vi "Configure Route Marker Signal.vi"(8 "error in (no error)":errorcluster, 10 "Route Marker Signal (0: M1)":i32(ring) items=["Marker 1", "Marker 2", "Marker 3", "Marker 4", "AUX29", "None"], 11 "VISA resource name":refnum<visa-resource-name>) -> (0 "error out":errorcluster, 3 "VISA resource name out":refnum<visa-resource-name>)   [LabVIEW 2018, in "Agilent PSG MXG Series.lvlib"]
doc: "Configures the marker single to be routed to the rear panel EVENT 1 connector.\n\n<b>Note:</b>\nIt is applicable for N5172B with <b>Option 653 or <b>Option 655</b>, N5182B with <b>Option 656</b> or <b>Option 657</b> only."
uses:
  Agilent PSG MXG Series.lvlib
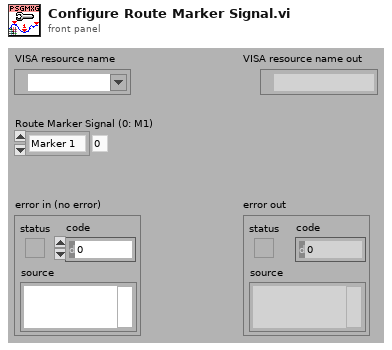
[diagram p1: front panel]
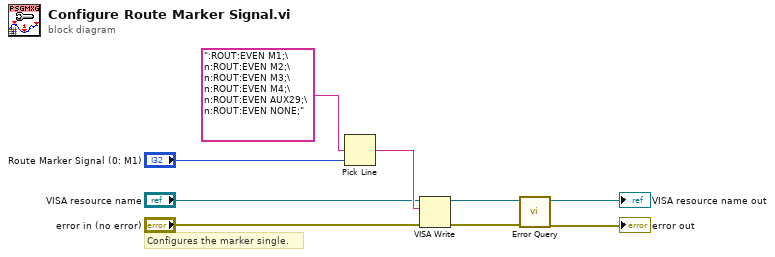
[diagram p0: block diagram]
diagram:
  # "Configures the marker single."
  n1 = Pick Line(multi-line string=":ROUT:EVEN M1;\n:ROUT:EVEN M2;\n:ROUT:EVEN M3;\n:ROUT:EVEN M4;\n:ROUT:EVEN AUX29;\n:ROUT:EVEN NONE;", line index="Route Marker Signal (0: M1)") -> (output string=w7:string)  [unwired: 1 in]
  n2 = VISA Write(VISA resource name="VISA resource name", write buffer=w7, error in (no error)="error in (no error)") -> (VISA resource name out=w4:refnum<visa-resource-name>, error out=w3:errorcluster)  [unwired: 1 out]
  n3 = call "Error Query.vi"("error in (no error)"=w3, "VISA resource name"=w4) -> ("error out"=→"error out":errorcluster, "VISA resource name out"=→"VISA resource name out":refnum<visa-resource-name>)  [unwired: 6 in, 2 out]
